vi "ArrayToExcel.vi"() -> ()   [LabVIEW 2020]
uses:
  <vilib>/Analysis/NI_AALBase.lvlib
panel:
  out "Waveform Graph":dbl[][](graph)
  out "F-format string":string[][](array[string])
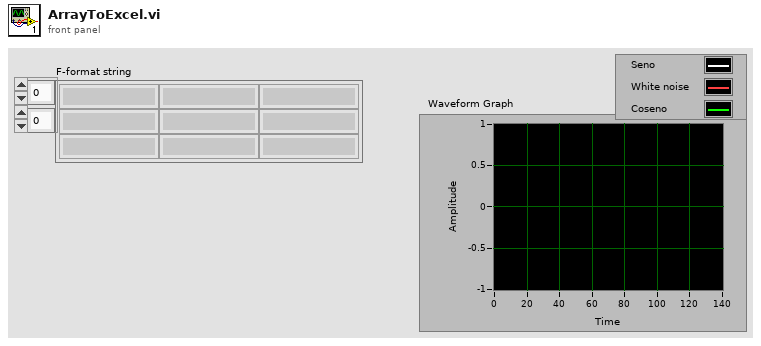
[diagram p1: front panel]
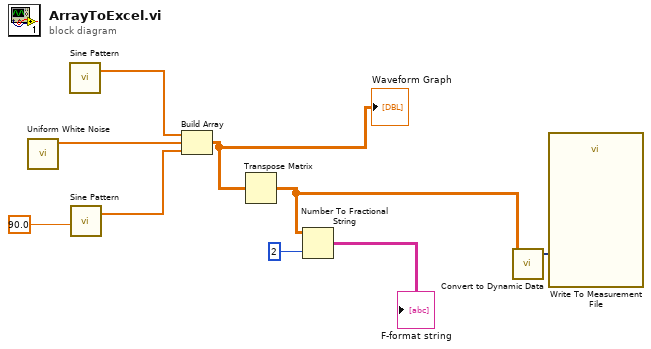
[diagram p0: block diagram]
diagram:
  n1 = call <vilib>:"Uniform White Noise.vi"() -> ("uniform white noise"=w8:dbl[])  [unwired: 10 in, 1 out]
  n2 = call <vilib>:"Sine Pattern.vi"() -> ("Sinusoidal Pattern"=w7:dbl[])  [unwired: 4 in, 1 out]
  n3 = call <vilib>:"Sine Pattern.vi"("phase(degrees)"=90.0) -> ("Sinusoidal Pattern"=w9:dbl[])  [unwired: 3 in, 1 out]
  n4 = Build Array(w7, w8, w9) -> (w2:dbl[][])
  "Waveform Graph" <- w2
  n5 = Transpose Matrix(1:w2) -> (0:w4:dbl[][])
  n6 = Number To Fractional String(number=w4, precision (6)=2) -> (F-format string=→"F-format string":string[][])  [unwired: 2 in]
  n7 = call "Convert to Dynamic Data"("2D Array"=w4) -> ("Dynamic Data Type"=w3:dynamicdata)  [unwired: 3 in]
  n8 = call "Write To Measurement File"("Signals"=w3) -> ()  [unwired: 16 in, 3 out]
